vi "getVideo.vi"(8 "error in (no error)":errorcluster, 10 "Video Id":string, 11 "YoutubeCacheProxy in":refnum<class "YoutubeCacheProxy.lvclass">) -> (0 "error out":errorcluster, 2 "Video":refnum<class "Video.lvclass">, 3 "YoutubeCacheProxy out":refnum<class "YoutubeCacheProxy.lvclass">)   [LabVIEW 2017, in "YoutubeCacheProxy.lvclass"]
uses:
  YoutubeCacheProxy.lvclass
  Video Class/Video.lvclass
  YoutubeCacheProxy.lvclass/YoutubeCacheProxy.ctl
  Video Class/Video.lvclass/Video.ctl
  Globals/ConsoleOut.vi
  ThirdPartyYoutubeLib Class/ThirdPartyYoutubeLib.lvclass
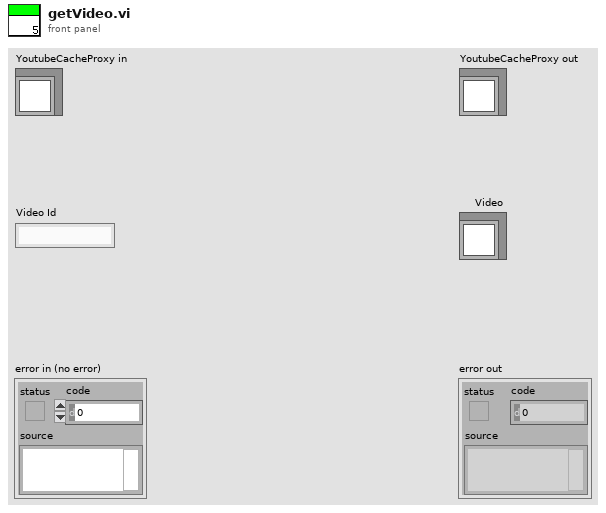
[diagram p1: front panel]
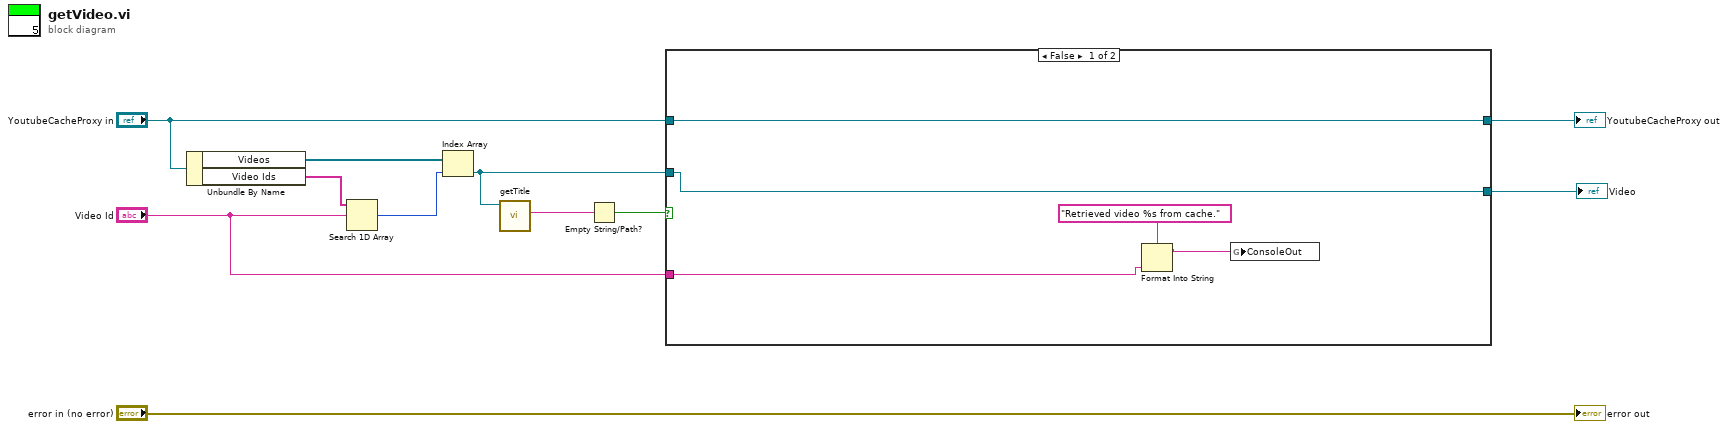
[diagram p0: block diagram]
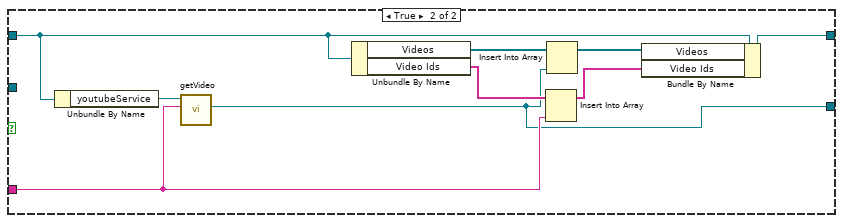
[diagram p2: hidden frame]
diagram:
  n1 = Unbundle By Name("YoutubeCacheProxy in") -> ("Videos"=w9:refnum<class "Video.lvclass">[], "Video Ids"=w10:string[])
  n2 = Search 1D Array(1D array=w10, element="Video Id") -> (index of element=w8:i32)  [unwired: 1 in]
  n3 = Index Array(array=w9, index=w8) -> (element=w1:refnum<class "Video.lvclass">)
  n4 = call "getTitle.vi"("Video in"=w1) -> ("title"=w7:string)  [unwired: 8 in, 2 out]
  n5 = Empty String/Path?(string/path=w7) -> (empty?=w4:bool)
  n6 = case shown="False" w4 {
    tunnel: "YoutubeCacheProxy in" -> [w16 w23]
    tunnel: [w16 w24] -> w5
    tunnel: "Video Id" -> [w12 w18]
    tunnel: [w15 w17] -> w2
    tunnel: w1 -> [w15 _]
    frame False {
      n7 = Format Into String(format string="Retrieved video %s from cache.", w12) -> (resulting string=w13:string)  [unwired: 2 in, 1 out]
      n8 = global write "ConsoleOut.vi" "ConsoleOut"(w13) -> ()
    }
    frame True {
      n9 = Unbundle By Name(w23) -> ("youtubeService"=w25:refnum<class "ThirdPartyYoutubeLib.lvclass">)
      n10 = call-dynamic "getVideo.vi"("Video Id"=w18, "ThirdPartyYoutubeLib in"=w25) -> ("Video"=w17:refnum<class "Video.lvclass">)  [unwired: 7 in, 2 out]
      n11 = Unbundle By Name(w23) -> ("Videos"=w22:refnum<class "Video.lvclass">[], "Video Ids"=w20:string[])
      n12 = Insert Into Array(array=w20, new element=w18) -> (w19:string[])  [unwired: 1 in]
      n13 = Insert Into Array(array=w22, new element=w17) -> (w21:refnum<class "Video.lvclass">[])  [unwired: 1 in]
      n14 = Bundle By Name(cluster=w23, "Videos"=w21, "Video Ids"=w19) -> (w24:refnum<class "YoutubeCacheProxy.lvclass">)
    }
  }
  "YoutubeCacheProxy out" <- w5
  "Video" <- w2
  "error out" <- "error in (no error)"
